vi "_Measurement Logic.vi"(8 "error in":errorcluster, 10 "measurement configuration":T2, 11 "measure call context in":refnum<class "Measure Call Context.lvclass">) -> (0 "error out":errorcluster, 2 "measurement results":T1, 3 "measure call context out":refnum<class "Measure Call Context.lvclass">)   [LabVIEW 2021, in "MeasurementServerTests.lvlib" / "Measurement Service Tests.lvlib" / "Continuous Counting Measurement.lvclass"]
uses:
  Continuous Counting Measurement.lvclass
  Runtime/Measurements/Measure Call Context/Measure Call Context.lvclass
  Measurement Configuration.ctl
  Measurement Results.ctl
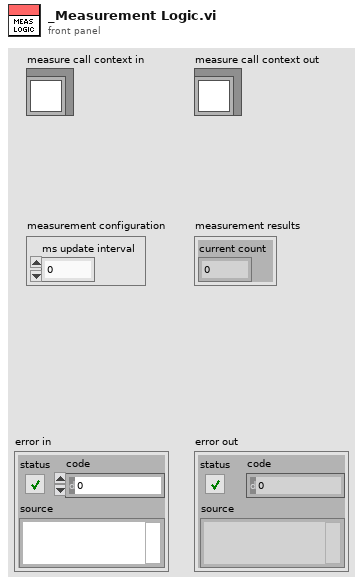
[diagram p1: front panel]
types:
  T1 = typedef "MeasurementServerTests.lvlib/Measurement Service Tests.lvlib/Continuous Counting Measurement.lvclass/Measurement Results.ctl" = cluster{"current count":i64}
  T2 = typedef "MeasurementServerTests.lvlib/Measurement Service Tests.lvlib/Continuous Counting Measurement.lvclass/Measurement Configuration.ctl" = cluster{"ms update interval":u32}
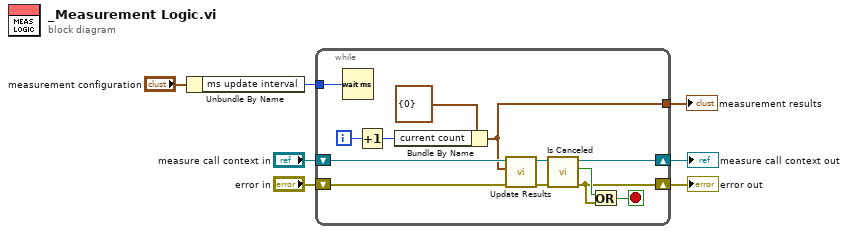
[diagram p0: block diagram]
diagram:
  n1 = Unbundle By Name("measurement configuration") -> ("ms update interval"=w2:u32)
  n2 = while {
    shift-right: [w20] -> w5
    shift-left: "measure call context in" -> [w11]
    shift-right: [w18] -> w3
    shift-left: "error in" -> [w14]
    tunnel: w2 -> [w12]
    tunnel: [w8] -> w1
    i -> [w16]
    stop <- w17 stop-if-true
    n3 = Wait (ms)(milliseconds to wait=w12) -> ()  [unwired: 1 out]
    n4 = Increment(x=w16) -> (x+1=w9:i32)
    n5 = Bundle By Name(cluster=T1 {"current count"=0} ("measurement results"), "current count"=w9) -> (w8:T1)
    n6 = call "Update Results.vi"("error in"=w14, "measurement results"=w8, "measure call context in"=w11) -> ("error out"=w13:errorcluster, "measure call context out"=w10:refnum<class "Measure Call Context.lvclass">)  [unwired: 7 in]
    n7 = call "Is Canceled.vi"("error in"=w13, "measure call context in"=w10) -> ("error out"=w18:errorcluster, "is canceled?"=w19:bool, "measure call context out"=w20:refnum<class "Measure Call Context.lvclass">)  [unwired: 7 in]
    n8 = Or(x=w19, y=w18) -> (x .or. y?=w17:bool)
  }
  "measure call context out" <- w5
  "error out" <- w3
  "measurement results" <- w1
